vi "Uninit.vi"(2 "Container State":T1, 3 "Display State":T2) -> ()   [LabVIEW 2017, in "XGaussfitGraph.lvlib" / "XGaussfitGraph.xctl"]
uses:
  XGaussfitGraph.xctl
  State.ctl
  <vilib>/_xctls/Container State.ctl
  <vilib>/_xctls/XControlSupport.lvlib
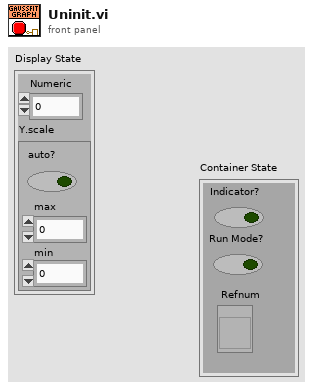
[diagram p1: front panel]
types:
  T1 = typedef "XControlSupport.lvlib/Container State.ctl" = cluster{"Indicator?":bool, "Run Mode?":bool, " Refnum":refnum<vi>}
  T2 = typedef "XGaussfitGraph.lvlib/XGaussfitGraph.xctl/State.ctl" = cluster{"Numeric":dbl, "Y.scale":cluster{"auto?":bool, "max":dbl, "min":dbl}}
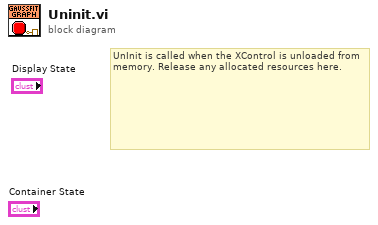
[diagram p0: block diagram]
diagram:
  # "UnInit is called when the XControl is unloaded from memory. Release any allocated resources here."
